vi "Sub_ParseStringIntoDoubleArray.vi"(2 "Received string":string, 3 "Number of active sensors":i16) -> (0 "Output data":dbl[](array[numeric]), 1 "Error array":bool[](array[boolean]))   [LabVIEW 2021]
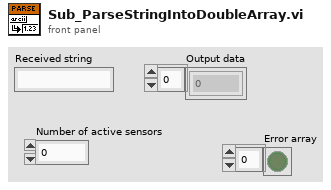
[diagram p1: front panel]
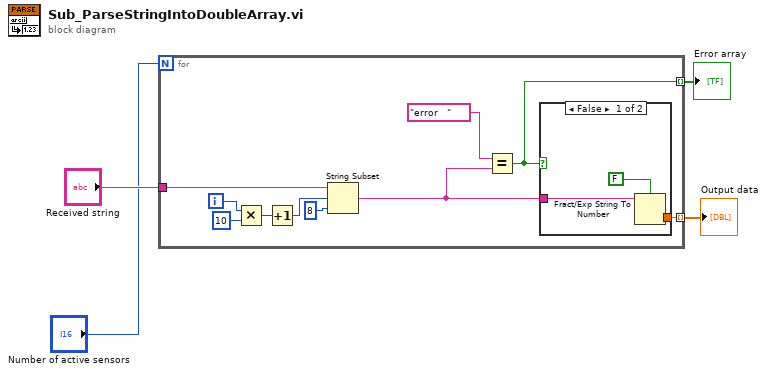
[diagram p0: block diagram]
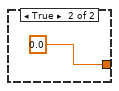
[diagram p2: hidden frame]
diagram:
  n1 = for {
    N: "Number of active sensors" -> [_]
    tunnel: "Received string" -> [w8]
    tunnel: [w9] -> w3 mode=indexing
    tunnel: [w5] -> w1 mode=indexing
    i -> [w13]
    n2 = Multiply(x=w13, y=10) -> (x*y=w11:i32)
    n3 = Increment(x=w11) -> (x+1=w10:i32)
    n4 = String Subset(string=w8, offset (0)=w10, length (rest)=8 ("length (rest)")) -> (substring=w6:string)
    n5 = Equal?(x="error   ", y=w6) -> (x = y?=w5:bool)
    n6 = case shown="False" w5 {
      tunnel: [w16 0.0] -> w9
      tunnel: w6 -> [w15 _]
      frame False {
        n7 = Fract/Exp String To Number(use system decimal point (T)=FALSE, string=w15) -> (number=w16:dbl)  [unwired: 2 in, 1 out]
      }
      frame True {
      }
    }
  }
  "Output data" <- w3
  "Error array" <- w1
